vi "Boolean Toggle.vi"(1 "Input":bool) -> (0 "Output":bool)   [LabVIEW 2013]
doc: "Changes a standard boolean input to a toggled boolean output."
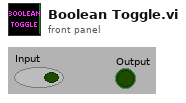
[diagram p1: front panel]
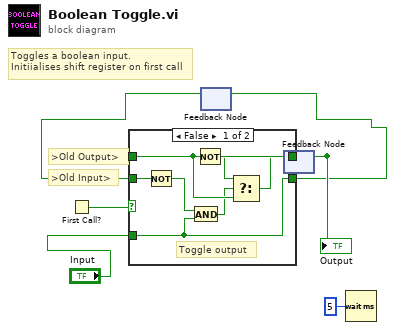
[diagram p0: block diagram]
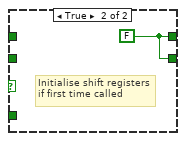
[diagram p2: hidden frame]
diagram:
  # ">Old Input>"
  # ">Old Output>"
  # "Toggles a boolean input.\nInitiialises shift register on first call"
  n1 = First Call?() -> (First Call?: T/F=w7:bool)
  n2 = feedback #1() -> (w1:bool)  [unwired: 1 in]
  n3 = feedback #2() -> (w3:bool)  [unwired: 1 in]
  "Output" <- w3
  n4 = case shown="False" w7 {
    tunnel: [w13 w15] -> w4
    tunnel: w3 -> [w12 _]
    tunnel: w1 -> [w8 _]
    tunnel: "Input" -> [w9 _]
    tunnel: [w9 w15] -> w2
    frame False {
      # "Toggle output"
      n5 = Not(x=w8) -> (.not. x?=w11:bool)
      n6 = And(x=w11, y=w9) -> (x .and. y?=w10:bool)
      n7 = Not(x=w12) -> (.not. x?=w14:bool)
      n8 = Select(t=w14, s=w10, f=w12) -> (s? t:f=w13:bool)
    }
    frame True {
      w15 = FALSE
      # "Initialise shift registers\nif first time called"
    }
  }
  n9 = feedback-in #1(w2) -> ()
  n10 = feedback-in #2(w4) -> ()
  n11 = Wait (ms)(milliseconds to wait=u32 5) -> ()  [unwired: 1 out]
